vi "Choreo_Util_AddTrajFileExtension.vi"(11 "FileName in":string) -> (3 "FileName out":string)   [LabVIEW 2019, in "ChoreoLib.lvlib"]
doc: "Add the .traj file extention, if missing, to the passed file name.\n\nInput:\n - filenamein - string - Filename string to check for extension and add if needed.\n\nOutput:\n - filenameout - string - modified filename"
uses:
  ChoreoLib.lvlib
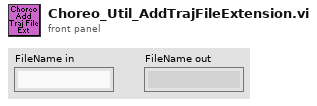
[diagram p1: front panel]
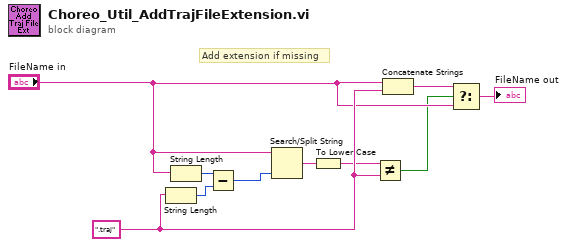
[diagram p0: block diagram]
diagram:
  w10 = ".traj" ("y")
  # "Add extension if missing"
  n1 = String Length(string=w10) -> (length=w9:i32)
  n2 = String Length(string="FileName in") -> (length=w1:i32)
  n3 = Subtract(x=w1, y=w9) -> (x-y=w2:i32)
  n4 = Search/Split String(string="FileName in", offset (0)=w2) -> (match + rest of string=w3:string)  [unwired: 1 in, 2 out]
  n5 = To Lower Case(string=w3) -> (all lower case string=w4:string)
  n6 = Not Equal?(x=w4, y=w10) -> (x != y?=w5:bool)
  n7 = Concatenate Strings("FileName in", w10) -> (w6:string)
  n8 = Select(t=w6, s=w5, f="FileName in") -> (s? t:f=→"FileName out":string)
